vi "to Array.vi"(8 "error in (no error)":errorcluster, 11 "Sweep Output in":refnum<class "Sweep Output.lvclass">) -> (0 "error out":errorcluster, 2 "Output values":dbl[](array[numeric]) format="%#_10p", 3 "Sweep Output out":refnum<class "Sweep Output.lvclass">)   [LabVIEW 2016, in "Sweep Output.lvclass"]
uses:
  Sweep Output.lvclass
  Sweep Output.lvclass/Sweep Output.ctl
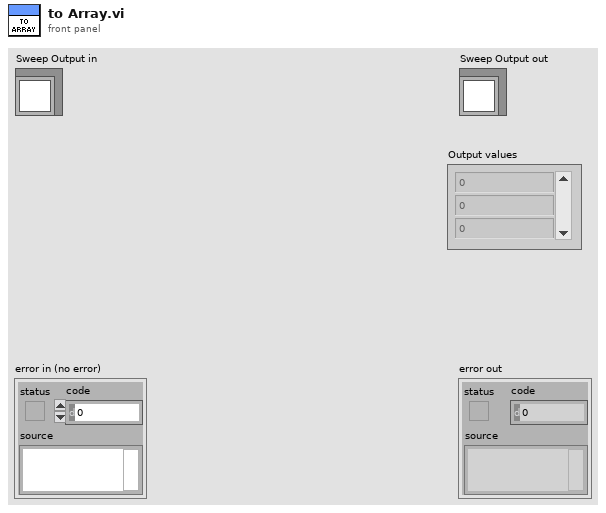
[diagram p1: front panel]
types:
  T1 = typedef "Increment mode.ctl" = enum16{"Linear", "Square root", "Square", "Log", "Exponent"}
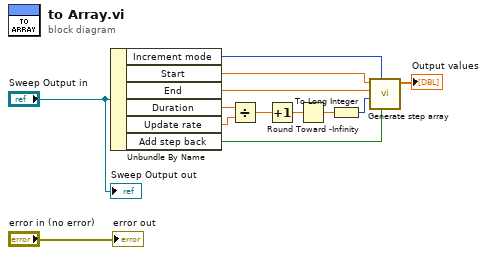
[diagram p0: block diagram]
diagram:
  n1 = Unbundle By Name("Sweep Output in") -> ("Increment mode"=w9:T1, "Start"=w13:dbl, "End"=w12:dbl, "Duration"=w11:dbl, "Update rate"=w10:dbl, "Add step back"=w8:bool)
  n2 = Divide(x=w11, y=w10) -> (x/y=w2:dbl)
  n3 = Increment(x=w2) -> (x+1=w3:dbl)
  n4 = Round Toward -Infinity(1:w3) -> (0:w4:dbl)
  n5 = To Long Integer(number=w4) -> (32bit integer=w1:i32)
  n6 = call "Generate step array.vi"("Add step back"=w8, "Increment mode"=w9, "Number of steps"=w1, "End"=w12, "Start"=w13) -> ("Steps"=→"Output values":dbl[])  [unwired: 6 in]
  "error out" <- "error in (no error)"
  "Sweep Output out" <- "Sweep Output in"
